vi "writeI32.vi"(8 "error in (no error)":errorcluster, 10 "Data":i32, 11 "II32Control in":refnum<class "II32Control.lvclass">) -> (0 "error out":errorcluster, 3 "II32Control out":refnum<class "II32Control.lvclass">)   [LabVIEW 2015, in "RTFPGA.lvlib" / "II32Control.lvclass"]
uses:
  II32Control.lvclass
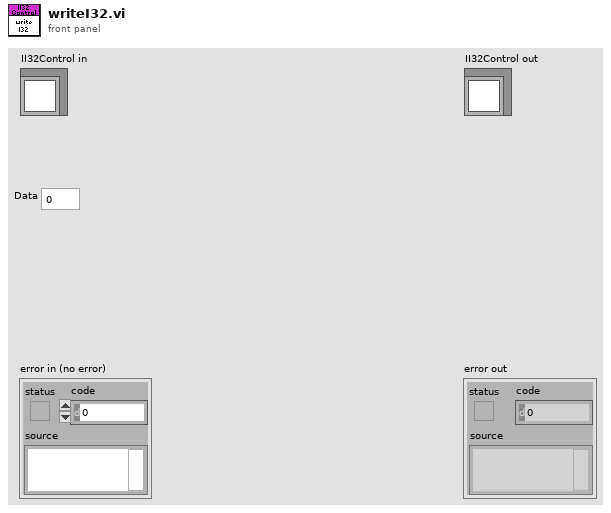
[diagram p1: front panel]
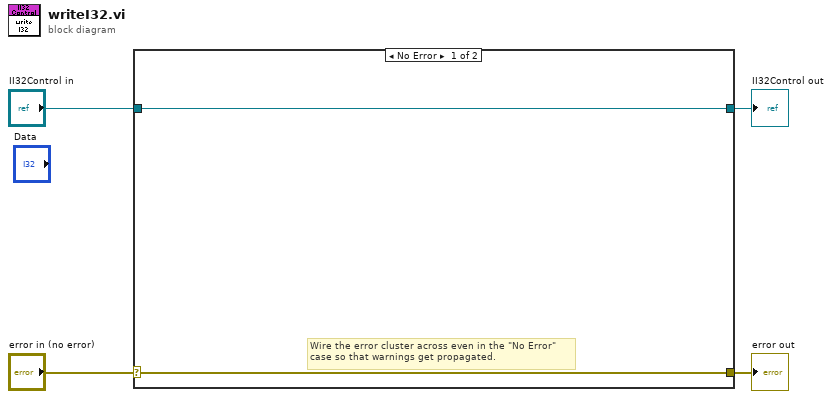
[diagram p0: block diagram]
diagram:
  n1 = case shown="No Error" "error in (no error)" {
    selector: "error in (no error)" -> [w5 w8]
    tunnel: [w5 w8] -> w3
    tunnel: [w6 w7] -> w1
    tunnel: "II32Control in" -> [w6 w7]
    frame No Error {
      # "Wire the error cluster across even in the \"No Error\"\ncase so that warnings get propagated."
    }
    frame Error {
    }
  }
  "error out" <- w3
  "II32Control out" <- w1
